vi "Initialise Cubes.vi"(8 "error in (no error)":errorcluster, 10 "Number Of Cubes":i32=10, 11 "Resource Directory":path) -> (0 "error out":errorcluster, 3 "Cubes":T1[](array[typedef]) {"Triangles"."Vertex 3"."UV"."v" min=0 max=1 step=0.1; "Triangles"."Vertex 3"."UV"."u" min=0 max=1 step=0.1; "Triangles"."Vertex 2"."UV"."v" min=0 max=1 step=0.1; "Triangles"."Vertex 2"."UV"."u" min=0 max=1 step=0.1; "Triangles"."Vertex 1"."UV"."v" min=0 max=1 step=0.1; "Triangles"."Vertex 1"."UV"."u" min=0 max=1 step=0.1})   [LabVIEW 2020, in "Scene.lvclass"]
uses:
  Scene.lvclass
  Scene.lvclass/Scene.ctl
  Graphics/Libraries/3D/3D.lvlib
  Graphics/Libraries/3D/Vector 3D.ctl
  Graphics/Libraries/3D/Transform.ctl
  <vilib>/numeric/Random Number (Range) DBL.vi
  Graphics/Libraries/3D/Object.ctl
  Graphics/Libraries/Raster/UV.ctl
  Graphics/Libraries/Raster/Raster.lvlib
  Graphics/Libraries/3D/Vertex.ctl
  Graphics/Libraries/3D/Triangle.ctl
  Graphics/Libraries/Raster/Rectangle Dimensions.ctl
  Graphics/Libraries/Raster/Texture.ctl
  Graphics/Libraries/3D/Material.ctl
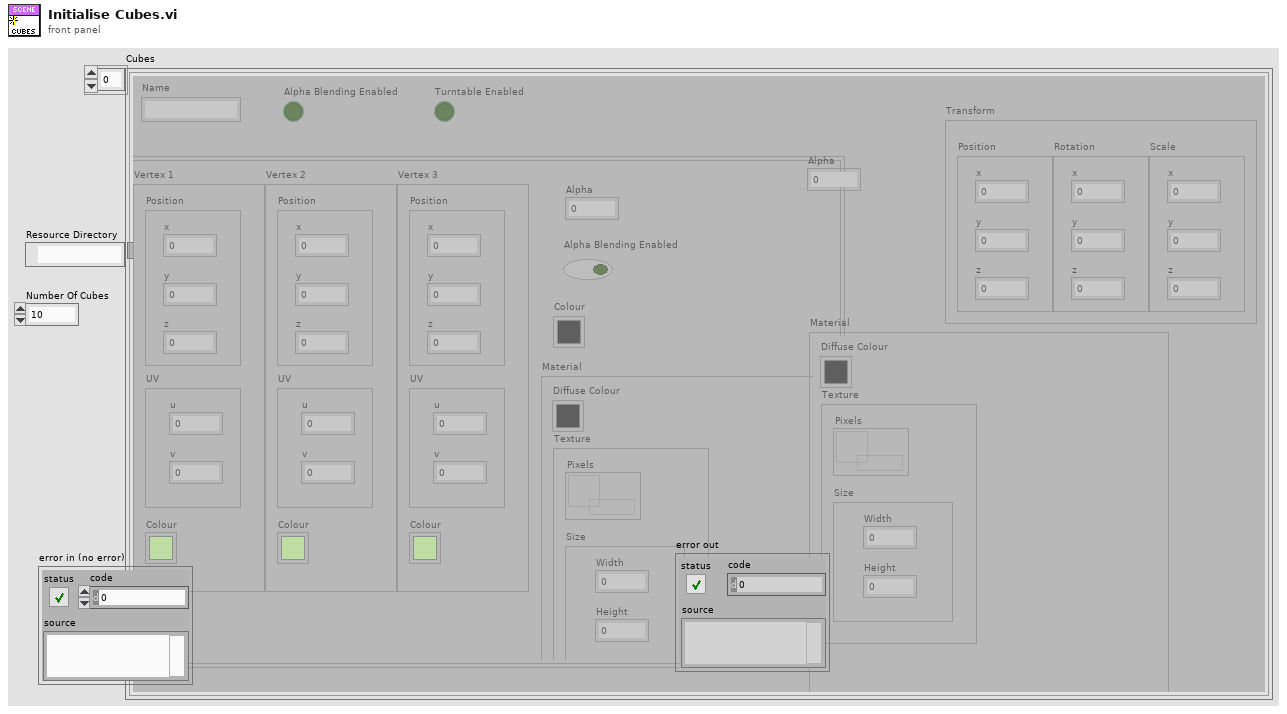
[diagram p1: front panel]
types:
  T1 = typedef "3D.lvlib/Object.ctl" = cluster{"Triangles":T2[], "Transform":T9, "Name":string, "Alpha Blending Enabled":bool, "Alpha":dbl, "Turntable Enabled":bool, "Material":T6}
  T2 = typedef "3D.lvlib/Triangle.ctl" = cluster{"Vertex 1":T3, "Vertex 2":T3, "Vertex 3":T3, "Alpha":dbl, "Alpha Blending Enabled":bool, "Colour":u32, "Material":T6}
  T3 = typedef "3D.lvlib/Vertex.ctl" = cluster{"Position":T4, "UV":T5, "Colour":u32}
  T4 = typedef "3D.lvlib/Vector 3D.ctl" = cluster{"x":sgl, "y":sgl, "z":sgl}
  T5 = typedef "Raster.lvlib/UV.ctl" = cluster{"u":sgl, "v":sgl}
  T6 = typedef "3D.lvlib/Material.ctl" = cluster{"Diffuse Colour":u32, "Texture":T7}
  T7 = typedef "Raster.lvlib/Texture.ctl" = cluster{"Pixels":refnum<data-value>, "Size":T8}
  T8 = typedef "Raster.lvlib/Rectangle Dimensions.ctl" = cluster{"Width":u32, "Height":u32}
  T9 = typedef "3D.lvlib/Transform.ctl" = cluster{"Position":T4, "Rotation":T4, "Scale":T4}
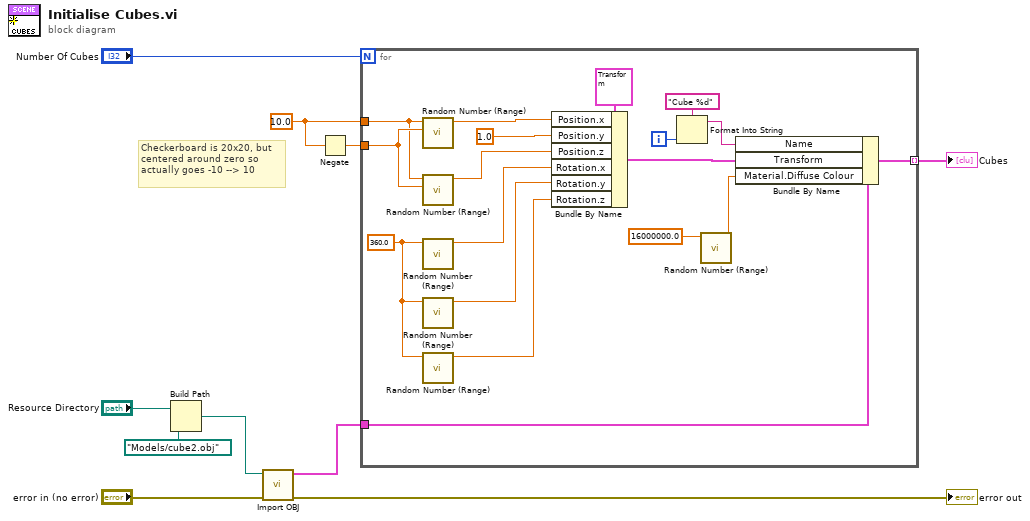
[diagram p0: block diagram]
diagram:
  w5 = 10.0 ("upper bound (100)")
  # "Checkerboard is 20x20, but centered around zero so actually goes -10 --> 10"
  n1 = Build Path(base path="Resource Directory", name or relative path=path "Models/cube2.obj") -> (appended path=w8:path)
  n2 = call "Import OBJ.vi"("error in (no error)"="error in (no error)", "Object"=w8) -> ("error out"=→"error out":errorcluster, "Object"=w10:T1)  [unwired: 8 in]
  n3 = Negate(x=w5) -> (-x=w4:dbl)
  n4 = for {
    N: "Number Of Cubes" -> [_]
    tunnel: w10 -> [w28]
    tunnel: [w24] -> w6 mode=indexing
    tunnel: w5 -> [w17]
    tunnel: w4 -> [w18]
    i -> [w21]
    w13 = 360.0 ("upper bound (100)")
    n5 = call-poly <vilib>:"Random Number (Range).vi"("lower bound (0)"=w18, "upper bound (100)"=w17) -> ("number"=w20:dbl)  [unwired: 9 in]
    n6 = call-poly <vilib>:"Random Number (Range).vi"("lower bound (0)"=w18, "upper bound (100)"=w17) -> ("number"=w19:dbl)  [unwired: 9 in]
    n7 = call-poly <vilib>:"Random Number (Range).vi"("upper bound (100)"=w13) -> ("number"=w14:dbl)  [unwired: 10 in]
    n8 = call-poly <vilib>:"Random Number (Range).vi"("upper bound (100)"=w13) -> ("number"=w12:dbl)  [unwired: 10 in]
    n9 = call-poly <vilib>:"Random Number (Range).vi"("upper bound (100)"=w13) -> ("number"=w11:dbl)  [unwired: 10 in]
    n10 = Bundle By Name(cluster=T9 {"Position"={"x"=2.0, "y"=1.0, "z"=-5.0}, "Rotation"={"x"=0.0, "y"=0.0, "z"=0.0}, "Scale"={"x"=0.0, "y"=0.0, "z"=0.0}} ("Transform"), "Position.x"=w20, "Position.y"=sgl 1.0, "Position.z"=w19, "Rotation.x"=w14, "Rotation.y"=w12, "Rotation.z"=w11) -> (w26:T9)
    n11 = Format Into String(format string="Cube %d" ("Name"), w21) -> (resulting string=w22:string)  [unwired: 2 in, 1 out]
    n12 = call-poly <vilib>:"Random Number (Range).vi"("upper bound (100)"=16000000.0) -> ("number"=w15:dbl)  [unwired: 10 in]
    n13 = Bundle By Name(cluster=w28, "Name"=w22, "Transform"=w26, "Material.Diffuse Colour"=w15) -> (w24:T1)
  }
  "Cubes" <- w6
